vi "Calibrate.vi"(8 "error in (no error)":errorcluster, 11 "Axsun_1310_SS in":refnum<class "Axsun_1310_SS.lvclass">) -> (0 "error out":errorcluster, 3 "Axsun_1310_SS out":refnum<class "Axsun_1310_SS.lvclass">)   [LabVIEW 2015, in "Axsun_1310_SS.lvclass"]
uses:
  Axsun_1310_SS.lvclass
  Laser.lvclass
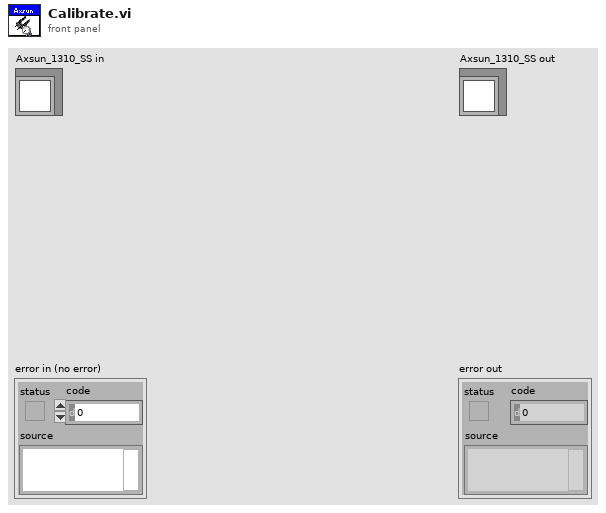
[diagram p1: front panel]
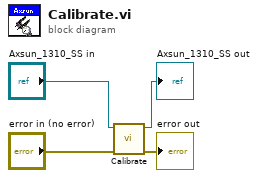
[diagram p0: block diagram]
diagram:
  n1 = call-parent "Calibrate.vi"("error in (no error)"="error in (no error)", "Laser in"="Axsun_1310_SS in") -> ("error out"=→"error out":errorcluster, "Laser out"=→"Axsun_1310_SS out":refnum<class "Axsun_1310_SS.lvclass">)  [unwired: 8 in]
